vi "simple wait func.vi"(11 "parameters":variant) -> (1 "error":errorcluster, 2 "data":variant, 3 "data ID":string)   [LabVIEW 2013]
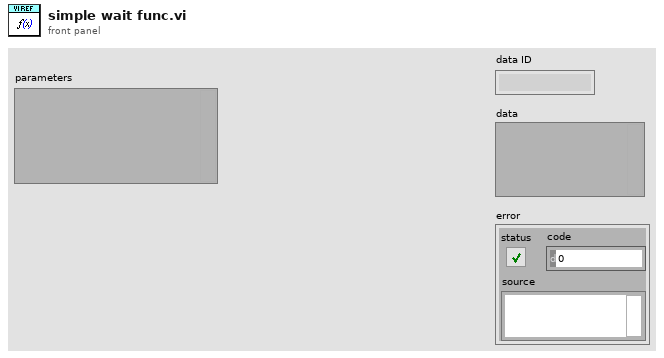
[diagram p1: front panel]
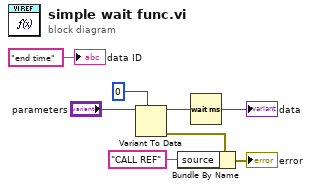
[diagram p0: block diagram]
diagram:
  n1 = Variant To Data(type=u32 0 ("milliseconds to wait"), Variant="parameters") -> (data=w5:u32, error out=w7:errorcluster)  [unwired: 1 in]
  n2 = Bundle By Name(cluster=w7, "source"="CALL REF") -> (→"error":errorcluster)
  n3 = Wait (ms)(milliseconds to wait=w5) -> (millisecond timer value=→"data":u32)
  "data ID" <- "end time" ("data ID")
